vi "Get Controller.vi"(11 "Processing in":refnum<class "Processing.lvclass">) -> (2 "Controller":refnum<class "Controller.lvclass">, 3 "Processing out":refnum<class "Processing.lvclass">)   [LabVIEW 2020, in "HTTP Server.lvlib" / "Processing.lvclass"]
uses:
  Processing.lvclass
  Controller/Controller.lvclass
  Processing.lvclass/Processing.ctl
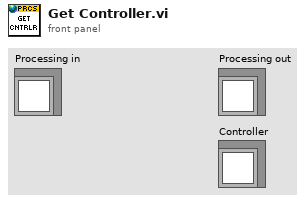
[diagram p1: front panel]
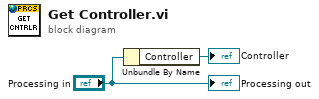
[diagram p0: block diagram]
diagram:
  n1 = Unbundle By Name("Processing in") -> ("Controller"=→"Controller":refnum<class "Controller.lvclass">)
  "Processing out" <- "Processing in"
